vi "Keep Array Size - Array.vi"(10 "Size":i32, 11 "Array In":dbl[](array[numeric])) -> (3 "Array Out":dbl[](array[numeric]))   [LabVIEW 2021]
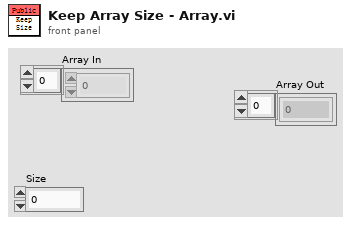
[diagram p1: front panel]
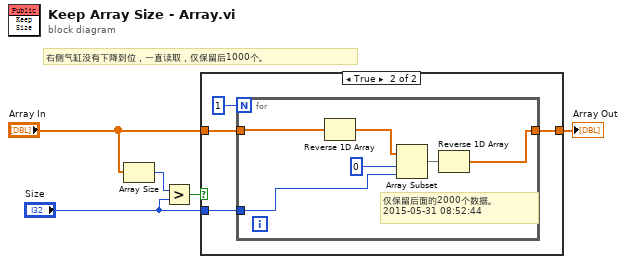
[diagram p0: block diagram]
diagram:
  # "右侧气缸没有下降到位，一直读取，仅保留后1000个。"
  n1 = Array Size(array="Array In") -> (size(s)=w4:i32)
  n2 = Greater?(x=w4, y="Size") -> (0:w5:bool)
  n3 = case shown="True" w5 {
    tunnel: "Array In" -> [w6 w9]
    tunnel: [w6 w10] -> w1
    tunnel: "Size" -> [_ w8]
    frame False {
    }
    frame True {
      n4 = for {
        N: 1 -> [_]
        tunnel: w9 -> [w12]
        tunnel: [w11] -> w10
        tunnel: w8 -> [w13]
        # "仅保留后面的2000个数据。\n2015-05-31 08:52:44"
        n5 = Reverse 1D Array(array=w12) -> (reversed array=w16:dbl[])
        n6 = Array Subset(array=w16, index=0, length=w13) -> (w14:dbl[])
        n7 = Reverse 1D Array(array=w14) -> (reversed array=w11:dbl[])
      }
    }
  }
  "Array Out" <- w1
